vi "Filter Empty Lines.vi"(0 "Functions in":T1[](array[typedef]), 11 "error in (no error)":errorcluster) -> (4 "Functions":T1[](array[typedef]), 15 "error out":errorcluster)   [LabVIEW 2016]
uses:
  Line Details.ctl
  <vilib>/Utility/error.llb/whitespace.ctl
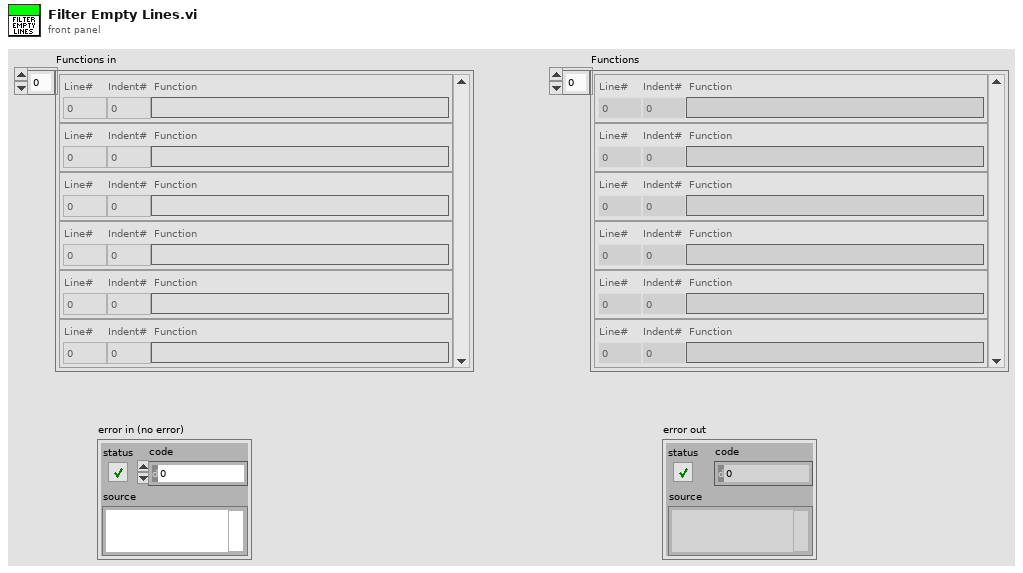
[diagram p1: front panel]
types:
  T1 = typedef "Line Details.ctl" = cluster{"Line#":i64, "Indent#":i64, "Function":string}
  T2 = typedef "whitespace.ctl" = u16
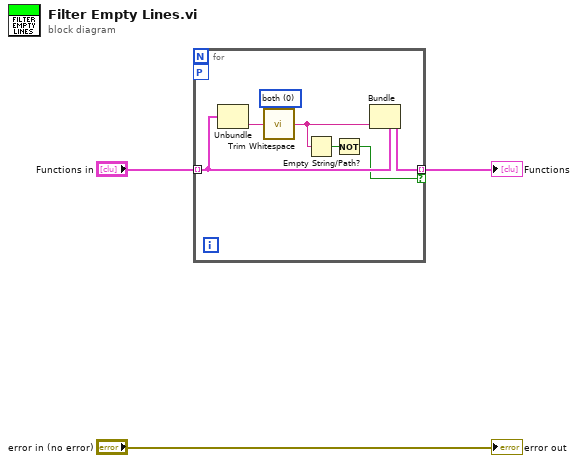
[diagram p0: block diagram]
diagram:
  n1 = for {
    tunnel: "Functions in" -> [w8] mode=indexing
    tunnel: [w5] -> w1 mode=indexing if=w4
    workers-P: _ -> [_]
    w9 = T2 0 items=["both", "start of string", "end of string"] ("location (both)")
    n2 = Unbundle(w8) -> ("Function"=w7:string)  [unwired: 2 out]
    n3 = call <vilib>:"Trim Whitespace.vi"("string"=w7, "location (both)"=w9) -> ("trimmed string"=w6:string)
    n4 = Empty String/Path?(string/path=w6) -> (empty?=w10:bool)
    n5 = Not(x=w10) -> (.not. x?=w4:bool)
    n6 = Bundle(cluster=w8, "Function"=w6) -> (w5:T1)  [unwired: 2 in]
  }
  "Functions" <- w1
  "error out" <- "error in (no error)"
